vi "Write Semaphore.vi"(8 "error in (no error)":errorcluster, 10 "semaphore":T1, 11 "VariableManager in":refnum<class "VariableManager.lvclass">) -> (0 "error out":errorcluster, 3 "VariableManager out":refnum<class "VariableManager.lvclass">)   [LabVIEW 2013, in "VariableManager.lvclass"]
uses:
  VariableManager.lvclass
  VariableManager.lvclass/VariableManager.ctl
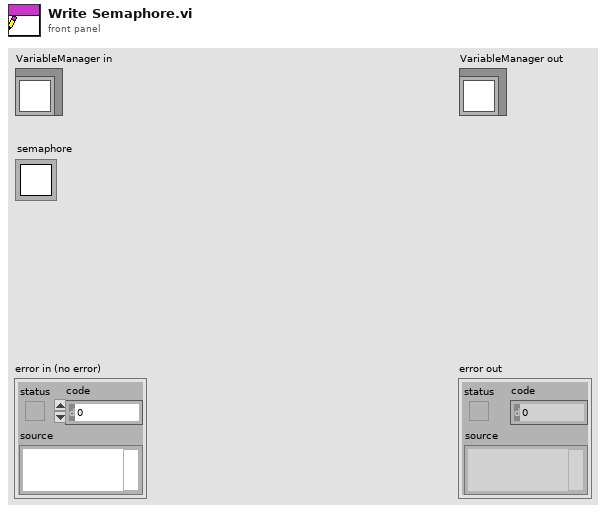
[diagram p1: front panel]
types:
  T1 = typedef "Semaphore RefNum" = refnum<k1>
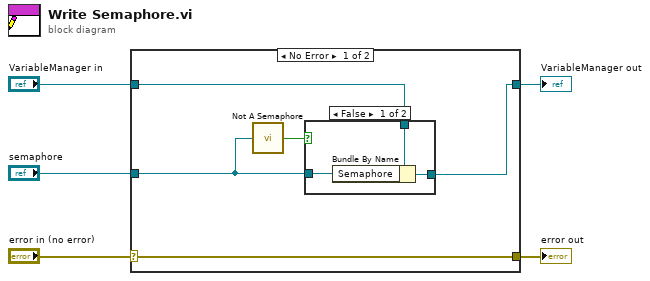
[diagram p0: block diagram]
diagram:
  n1 = case shown="No Error" "error in (no error)" {
    selector: "error in (no error)" -> [w10 w15]
    tunnel: [w10 w15] -> w4
    tunnel: [w8 w16] -> w2
    tunnel: "VariableManager in" -> [w9 w16]
    tunnel: "semaphore" -> [w7 _]
    frame No Error {
      n2 = call <vilib>:"Not A Semaphore.vi"("semaphore"=w7) -> ("not a semaphore"=w6:bool)
      n3 = case shown="False" w6 {
        tunnel: w9 -> [w13 w14]
        tunnel: [w12 w14] -> w8
        tunnel: w7 -> [w11 _]
        frame False {
          n4 = Bundle By Name(cluster=w13, "Semaphore"=w11) -> (w12:refnum<class "VariableManager.lvclass">)
        }
        frame True {
        }
      }
    }
    frame Error {
    }
  }
  "error out" <- w4
  "VariableManager out" <- w2
